vi "Settings_Variant_FGV.vi"(0 "Variant":variant, 1 "XML Path":path=path "D:/TEST.xml", 3 "error in (no error)":errorcluster, 4 "Command":enum16{"Read XML", "Set", "Get", "Write XML"}(ring)) -> (6 "Variant Output":variant, 7 "XML String Out":string, 9 "error out":errorcluster)   [LabVIEW 2015]
uses:
  <vilib>/NI/GXML/_subVIs/GXML SearchParser/Search Parser.vi
  <vilib>/NI/GXML/GXML.lvlib
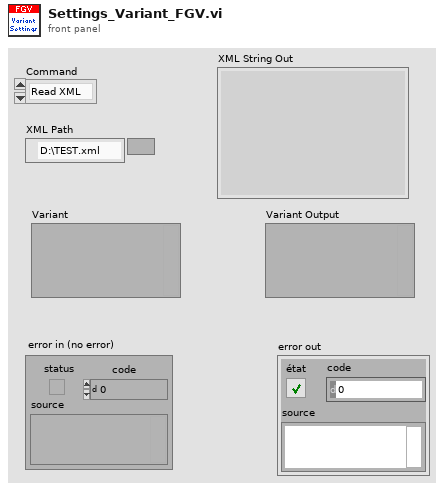
[diagram p1: front panel]
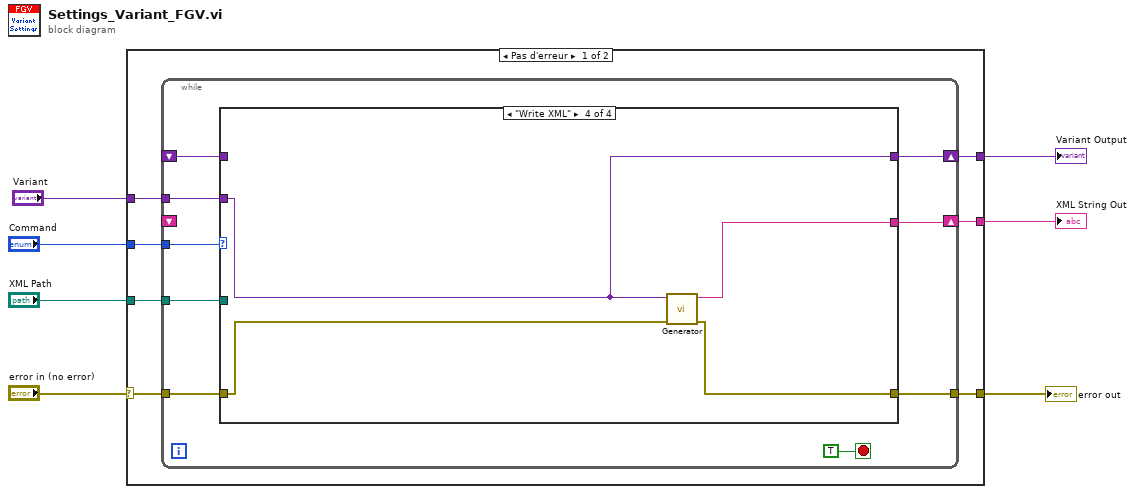
[diagram p0: block diagram]
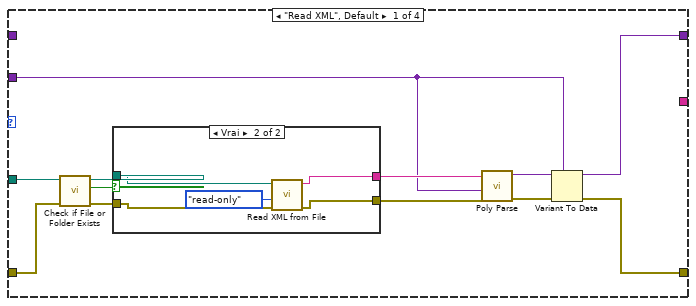
[diagram p2: hidden frame]
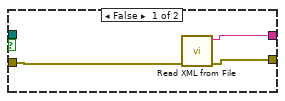
[diagram p3: hidden frame]
diagram:
  n1 = case shown="Pas d'erreur" "error in (no error)" {
    selector: "error in (no error)" -> [w12 w53]
    tunnel: "Command" -> [w14 _]
    tunnel: [w13 w52] -> w2
    tunnel: [w11 w53] -> w5
    tunnel: "XML Path" -> [w10 _]
    tunnel: "Variant" -> [w9 w52]
    tunnel: [w8 _] -> w1
    frame No Error {
      n2 = while {
        tunnel: w14 -> [w22]
        shift-right: [w20] -> w13
        shift-left: _ -> [w21]
        tunnel: w12 -> [w19]
        tunnel: [w18] -> w11
        tunnel: w10 -> [w17]
        tunnel: w9 -> [w16]
        shift-right: [w15] -> w8
        shift-left: _ -> [_]
        stop <- TRUE stop-if-true
        n3 = case shown="\"Write XML\"" w22 {
          tunnel: w21 -> [_ _ w47 _]
          tunnel: [w30 w44 w47 w48] -> w20
          tunnel: w19 -> [w32 w45 w46 w50]
          tunnel: [w28 w45 w46 w49] -> w18
          tunnel: w17 -> [w26 _ _ _]
          tunnel: w16 -> [w24 w44 _ w48]
          tunnel: [_ _ _ w51] -> w15
          frame "Read XML", Default {
            n4 = call <vilib>:"Check if File or Folder Exists.vi"("error in (no error)"=w32, "path"=w26) -> ("error out"=w35:errorcluster, "file or folder exists?"=w34:bool, "dup path"=w33:path)  [unwired: 7 in]
            n5 = case shown="Vrai" w34 {
              tunnel: w33 -> [_ w43]
              tunnel: w35 -> [w38 w41]
              tunnel: [w36 w42] -> w25
              tunnel: [w37 w40] -> w29
              frame False {
                n6 = call <vilib>:"Read XML from File.vi"("error in"=w38) -> ("error out"=w37:errorcluster, "XML String Out"=w36:string)  [unwired: 9 in]
              }
              frame True {
                n7 = call <vilib>:"Read XML from File.vi"("error in"=w41, "file access"=enum16{"read/write", "read-only", "write-only"}."read-only", "XML File Path"=w43) -> ("error out"=w40:errorcluster, "XML String Out"=w42:string)  [unwired: 7 in]
              }
            }
            n8 = call-poly <vilib>:"Poly Parse.vi"("error in"=w29, "TypeDesc"=w24, "XML String In"=w25) -> ("error out"=w27:errorcluster, "Parsed Data"=w31:variant)  [unwired: 7 in]
            n9 = Variant To Data(error in=w27, type=w24, Variant=w31) -> (data=w30:variant, error out=w28:errorcluster)
          }
          frame "Set" {
          }
          frame "Get" {
          }
          frame "Write XML" {
            n10 = call <vilib>:"Generator.vi"("error in"=w50, "Variant"=w48) -> ("error out"=w49:errorcluster, "XML String Out"=w51:string)  [unwired: 8 in]
          }
        }
      }
    }
    frame Error {
    }
  }
  "error out" <- w5
  "Variant Output" <- w2
  "XML String Out" <- w1
